vi "ControllerCore.vi"(8 "error in (no error)":errorcluster, 9 "FRC Joystick?":bool, 10 "JoystickDevRef":T1) -> (0 "error out":errorcluster, 3 "Driver controller":T3)   [LabVIEW 2014]
uses:
  <vilib>/Rock Robotics/WPI/Joystick/WPI_JoystickDevRef.ctl
  <vilib>/Rock Robotics/WPI/Joystick/WPI_JoystickDeviceEnum.ctl
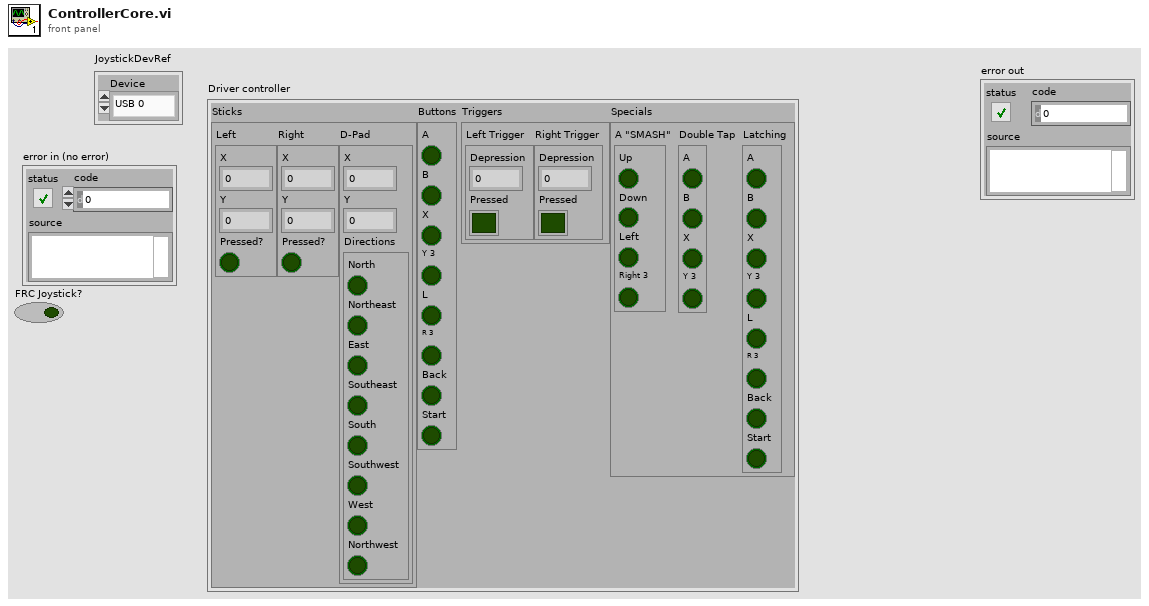
[diagram p1: front panel]
types:
  T1 = typedef "WPI_JoystickDevRef.ctl" = cluster{"Device":T2}
  T2 = typedef "WPI_JoystickDeviceEnum.ctl" = enum16{"USB 0", "USB 1", "USB 2", "USB 3", "USB 4", "USB 5"}
  T3 = cluster{"Sticks":cluster{"Left":cluster{"X":dbl, "Y":dbl, "Pressed?":bool}, "Right":cluster{"X":dbl, "Y":dbl, "Pressed?":bool}, "D-Pad":cluster{"X":dbl, "Y":dbl, "Directions":cluster{"North":bool, "Northeast":bool, "East":bool, "Southeast":bool, "South":bool, "Southwest":bool, "West":bool, "Northwest":bool}}}, "Buttons":cluster{"A":bool, "B":bool, "X":bool, "Y 3":bool, "L":bool, "R 3":bool, "Back":bool, "Start":bool}, "Triggers":cluster{"Left Trigger":cluster{"Depression":dbl, "Pressed":bool}, "Right Trigger":cluster{"Depression":dbl, "Pressed":bool}}, "Specials":cluster{"A \"SMASH\"":cluster{"Up":bool, "Down":bool, "Left":bool, "Right 3":bool}, "Double Tap":cluster{"A":bool, "B":bool, "X":bool, "Y 3":bool}, "Latching":cluster{"A":bool, "B":bool, "X":bool, "Y 3":bool, "L":bool, "R 3":bool, "Back":bool, "Start":bool}}}
  T4 = cluster{"Sticks":cluster{"Left":cluster{"X":dbl, "Y":dbl, "Pressed?":bool}, "Right":cluster{"X":dbl, "Y":dbl, "Pressed?":bool}, "D-Pad":cluster{"X":dbl, "Y":dbl, "Directions":cluster{"North":bool, "Northeast":bool, "East":bool, "Southeast":bool, "South":bool, "Southwest":bool, "West":bool, "Northwest":bool}}}, "Buttons":cluster{"A":bool, "B":bool, "X":bool, "Y 3":bool, "L":bool, "R 3":bool, "Back":bool, "Start":bool}, "Triggers":cluster{"Left Trigger":cluster{"Depression":dbl, "Pressed":bool}, "Right Trigger":cluster{"Depression":dbl, "Pressed":bool}}, "Specials":cluster{"L Stick \"SMASH\"":cluster{"A":bool, "B":bool, "X":bool, "Y 3":bool}, "Double Tap":cluster{"A":bool, "B":bool, "X":bool, "Y 3":bool}, "Latching":cluster{"A":bool, "B":bool, "X":bool, "Y 3":bool, "L":bool, "R 3":bool, "Back":bool, "Start":bool}}}
  T5 = cluster{"North":bool, "Northeast":bool, "East":bool, "Southeast":bool, "South":bool, "Southwest":bool, "West":bool, "Northwest":bool}
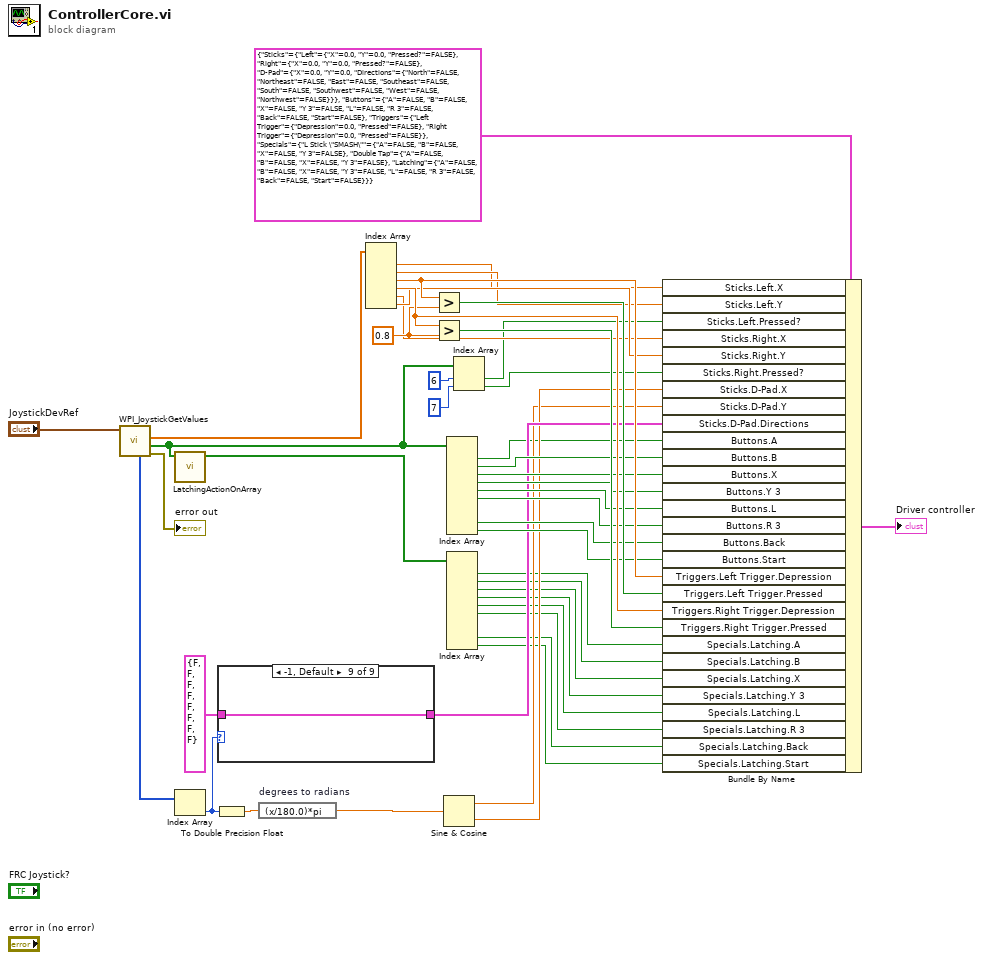
[diagram p0: block diagram]
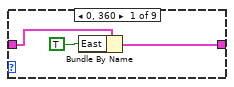
[diagram p2: hidden frame]
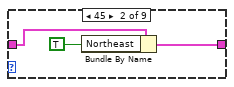
[diagram p3: hidden frame]
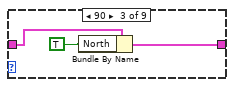
[diagram p4: hidden frame]
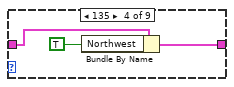
[diagram p5: hidden frame]
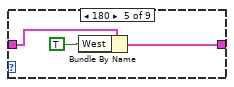
[diagram p6: hidden frame]
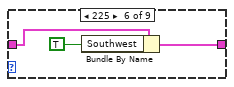
[diagram p7: hidden frame]
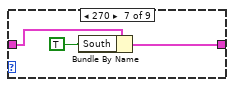
[diagram p8: hidden frame]
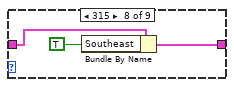
[diagram p9: hidden frame]
diagram:
  w43 = 0.8 ("y")
  n1 = call <vilib>:"WPI_JoystickGetValues.vi"("JoystickDevRef"="JoystickDevRef") -> ("error out"=→"error out":errorcluster, "Buttons"=w9:bool[], "Axes"=w16:dbl[], "POVs"=w23:i16[])  [unwired: 6 in, 1 out]
  n2 = call "LatchingActionOnArray.vi"("Array of booleans"=w9) -> ("Latched booleeans"=w10:bool[])  [unwired: 10 in]
  n3 = Index Array(array=w23) -> (element=w28:i16)  [unwired: 1 in]
  n4 = To Double Precision Float(number=w28) -> (double precision float=w24:dbl)
  n5 = case shown="-1, Default" w28 {
    tunnel: T5 {"North"=FALSE, "Northeast"=FALSE, "East"=FALSE, "Southeast"=FALSE, "South"=FALSE, "Southwest"=FALSE, "West"=FALSE, "Northwest"=FALSE} ("Sticks.D-Pad.Directions") -> [w47 w50 w53 w56 w59 w62 w65 w68 w69]
    tunnel: [w46 w49 w52 w55 w58 w61 w64 w67 w69] -> w30
    frame 0, 360 {
      n6 = Bundle By Name(cluster=w47, "East"=TRUE) -> (w46:T5)
    }
    frame 45 {
      n7 = Bundle By Name(cluster=w50, "Northeast"=TRUE ("East")) -> (w49:T5)
    }
    frame 90 {
      n8 = Bundle By Name(cluster=w53, "North"=TRUE ("East")) -> (w52:T5)
    }
    frame 135 {
      n9 = Bundle By Name(cluster=w56, "Northwest"=TRUE ("East")) -> (w55:T5)
    }
    frame 180 {
      n10 = Bundle By Name(cluster=w59, "West"=TRUE ("East")) -> (w58:T5)
    }
    frame 225 {
      n11 = Bundle By Name(cluster=w62, "Southwest"=TRUE ("East")) -> (w61:T5)
    }
    frame 270 {
      n12 = Bundle By Name(cluster=w65, "South"=TRUE ("East")) -> (w64:T5)
    }
    frame 315 {
      n13 = Bundle By Name(cluster=w68, "Southeast"=TRUE ("East")) -> (w67:T5)
    }
    frame -1, Default {
    }
  }
  n14 = expression code="(x/180.0)*pi" "degrees to radians"(w24) -> (w25:dbl)
  n15 = Index Array(array=w16) -> (element #1=w13:dbl, element #2=w17:dbl, element #3=w40:dbl, element #4=w44:dbl, element #5=w38:dbl, element #6=w39:dbl)  [unwired: 6 in]
  n16 = Greater?(x=w40, y=w43) -> (0:w41:bool)
  n17 = Greater?(x=w44, y=w43) -> (0:w42:bool)
  n18 = Sine & Cosine(0:w25) -> (1:w26:dbl, 2:w27:dbl)
  n19 = Index Array(array=w9) -> (element #1=w14:bool, element #2=w31:bool, element #3=w32:bool, element #4=w33:bool, element #5=w34:bool, element #6=w35:bool, element #9=w36:bool, element #10=w37:bool)  [unwired: 10 in, 2 out]
  n20 = Index Array(array=w10) -> (element #1=w8:bool, element #2=w7:bool, element #3=w6:bool, element #4=w5:bool, element #5=w4:bool, element #6=w3:bool, element #9=w2:bool, element #10=w1:bool)  [unwired: 10 in, 2 out]
  n21 = Index Array(array=w9, index #1=6 ("index"), index #2=7 ("index")) -> (element #1=w20:bool, element #2=w21:bool)
  n22 = Bundle By Name(cluster=T4 {"Sticks"={"Left"={"X"=0.0, "Y"=0.0, "Pressed?"=FALSE}, "Right"={"X"=0.0, "Y"=0.0, "Pressed?"=FALSE}, "D-Pad"={"X"=0.0, "Y"=0.0, "Directions"={"North"=FALSE, "Northeast"=FALSE, "East"=FALSE, "Southeast"=FALSE, "South"=FALSE, "Southwest"=FALSE, "West"=FALSE, "Northwest"=FALSE}}}, "Buttons"={"A"=FALSE, "B"=FALSE, "X"=FALSE, "Y 3"=FALSE, "L"=FALSE, "R 3"=FALSE, "Back"=FALSE, "Start"=FALSE}, "Triggers"={"Left Trigger"={"Depression"=0.0, "Pressed"=FALSE}, "Right Trigger"={"Depression"=0.0, "Pressed"=FALSE}}, "Specials"={"L Stick \"SMASH\""={"A"=FALSE, "B"=FALSE, "X"=FALSE, "Y 3"=FALSE}, "Double Tap"={"A"=FALSE, "B"=FALSE, "X"=FALSE, "Y 3"=FALSE}, "Latching"={"A"=FALSE, "B"=FALSE, "X"=FALSE, "Y 3"=FALSE, "L"=FALSE, "R 3"=FALSE, "Back"=FALSE, "Start"=FALSE}}} ("Driver controller 2"), "Sticks.Left.X"=w13, "Sticks.Left.Y"=w17, "Sticks.Left.Pressed?"=w20, "Sticks.Right.X"=w38, "Sticks.Right.Y"=w39, "Sticks.Right.Pressed?"=w21, "Sticks.D-Pad.X"=w27, "Sticks.D-Pad.Y"=w26, "Sticks.D-Pad.Directions"=w30, "Buttons.A"=w14, "Buttons.B"=w31, "Buttons.X"=w32, "Buttons.Y 3"=w33, "Buttons.L"=w34, "Buttons.R 3"=w35, "Buttons.Back"=w36, "Buttons.Start"=w37, "Triggers.Left Trigger.Depression"=w40, "Triggers.Left Trigger.Pressed"=w41, "Triggers.Right Trigger.Depression"=w44, "Triggers.Right Trigger.Pressed"=w42, "Specials.Latching.A"=w8, "Specials.Latching.B"=w7, "Specials.Latching.X"=w6, "Specials.Latching.Y 3"=w5, "Specials.Latching.L"=w4, "Specials.Latching.R 3"=w3, "Specials.Latching.Back"=w2, "Specials.Latching.Start"=w1) -> (→"Driver controller":T4)
